vi "ReadOhmsValue.vi"(8 "error in":errorcluster, 10 "nDelayValue":i32=15000, 11 "nScale":i32=5) -> (0 "error out":errorcluster, 1 "*pnChanSpanOffset":i32=3006, 2 "*pnChanZeroOffset":i32=2053, 3 "Return Code":i32, 5 "*pnOhmValue":i32=3005)   [LabVIEW 2015]
doc: "MEScope_ReadOhmsVal\nDescription:\nThis function will read the Ohms multimeter ADC offset.\nDetail:\nint MEScope_ReadOhmsVal (\nint nScale, \nint *pnOhmValue, \nint nDelayValue, \nint *pnChanZeroOffset,\nint *pnChanSpanOffset\n);\nParameters:\nint nScale - which scale to use (MM_OHMS_400 to MM_OHMS_4MEG)\n\nint *pnOhmValue - pointer to an integer, filled with the Ohms ADC count.\n\nint nDelayValue - A delay value in mS, based on the table below:\n\n G16 Values:\nScale 40 400 4 k 40 k 400 k 4 Meg\nDelay 100 100 100 500 2000 15000\n\nint * pnChanZeroOffset - pointer to an integer, filled with the zero offset calibration value for the requested scale. It can be NULL if the data isn't required.\n\nint * pnChanSpanOffset - pointer to an integer, filled with the span offset calibration value for the requested scale. It can be NULL if the data isn't required.\n\nReturn Values:\nThis function returns a 0 if the function completed successfully. A non-zero return code will indicate error. \nRemarks:\nG16 Scale definitions:\n#define M5_OHMS_40 0\n#define M5_OHMS_400 1\n#define M5_OHMS_4K 2\n#define M5_OHMS_40K 3\n#define M5_OHMS_400K 4\n#define M5_OHMS_4MEG 5\n\nSee Appendix 4 for details on converting ADC reading into a measurement.\nSerial Command packet: \nn/a"
uses:
  ScannerDiagDLL.dll
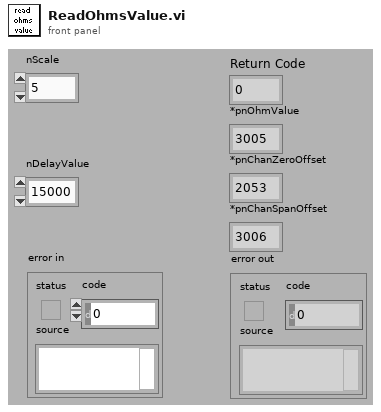
[diagram p1: front panel]
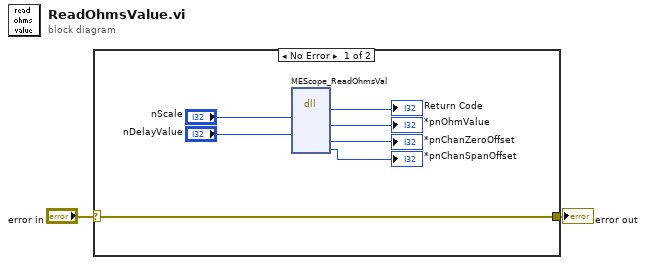
[diagram p0: block diagram]
diagram:
  n1 = case shown="No Error" "error in" {
    selector: "error in" -> [w3 w10]
    tunnel: [w3 w10] -> w1
    frame No Error {
      n2 = dll-call lib="C:/ModisEdge/Scope/Test Sequence/Code Modules/DLL/ScannerDiagDLL.dll" fn="MEScope_ReadOhmsVal"("nScale"="nScale", "nDelayValue"="nDelayValue") -> ("return type"=→"Return Code":i32, "pnOhmValue"=→"*pnOhmValue":i32, "pnChanZeroOffset"=→"*pnChanZeroOffset":i32, "pnChanSpanOffset"=→"*pnChanSpanOffset":i32)  [unwired: 8 in, 2 out]
    }
    frame Error {
    }
  }
  "error out" <- w1
